vi "SeqMgr.Update Controls.vi"(8 "error in (no error)":errorcluster, 11 "SeqMgr in":refnum<class "SeqMgr.lvclass">) -> (0 "error out":errorcluster, 3 "SeqMgr out":refnum<class "SeqMgr.lvclass">)   [LabVIEW 2024, in "EQMF.lvlib" / "SeqMgr.lvlib" / "SeqMgr.lvclass"]
uses:
  SeqMgr.lvclass
  SeqMgr.lvclass/SeqMgr.ctl
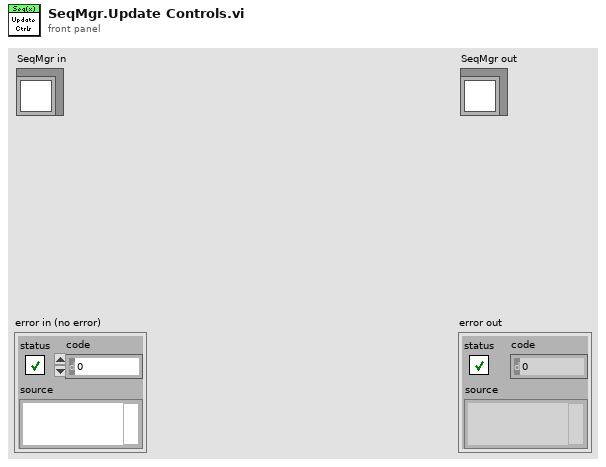
[diagram p1: front panel]
types:
  T1 = typedef "EQMF.lvlib/SeqMgr.lvlib/SeqMgr.Result State Enum.ctl" = enum16{"None", "Passing", "Failing", "PASS", "FAIL", "ABORT", "ERROR"}
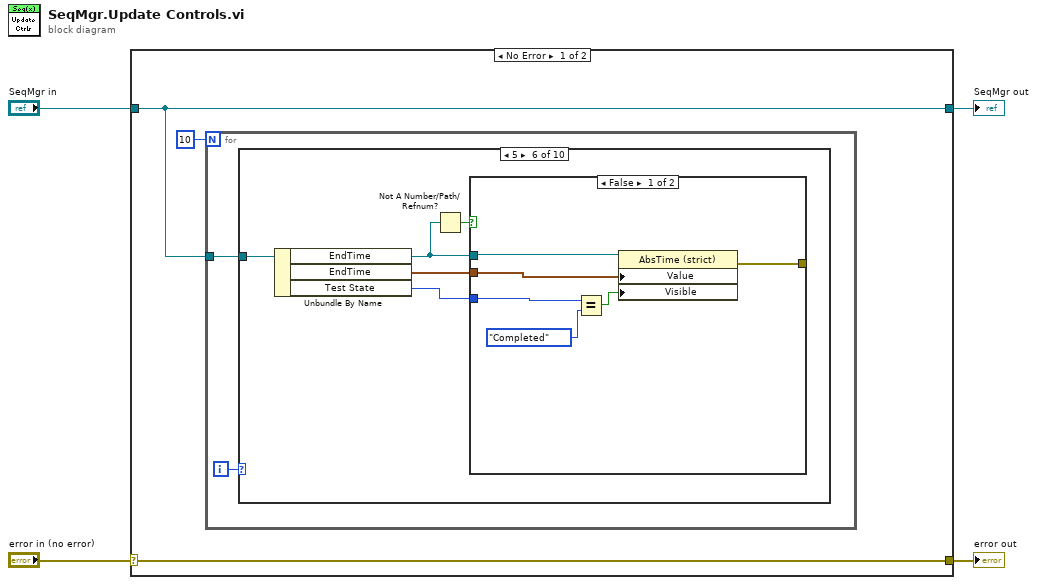
[diagram p0: block diagram]
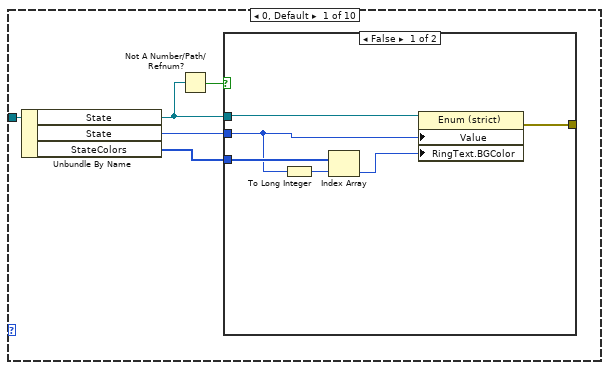
[diagram p2: hidden frame]
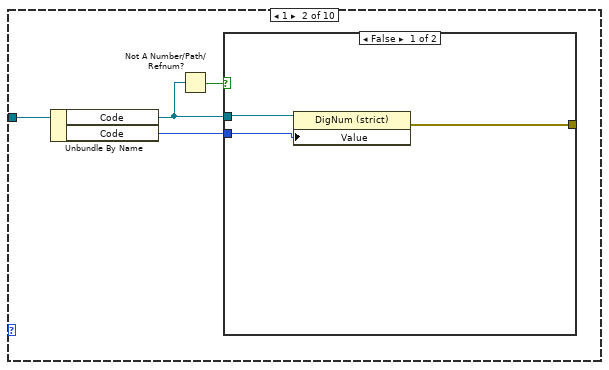
[diagram p4: hidden frame]
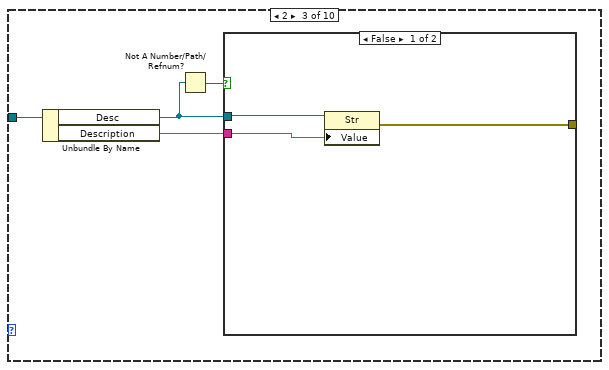
[diagram p6: hidden frame]
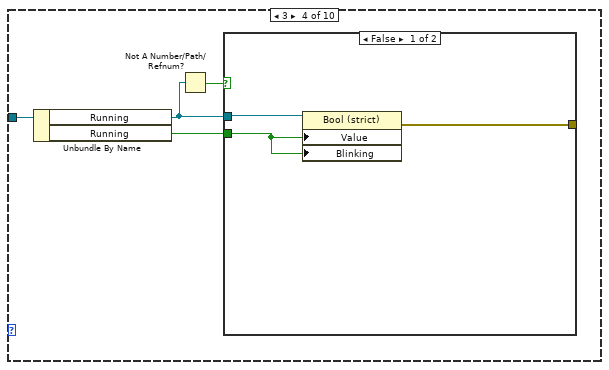
[diagram p8: hidden frame]
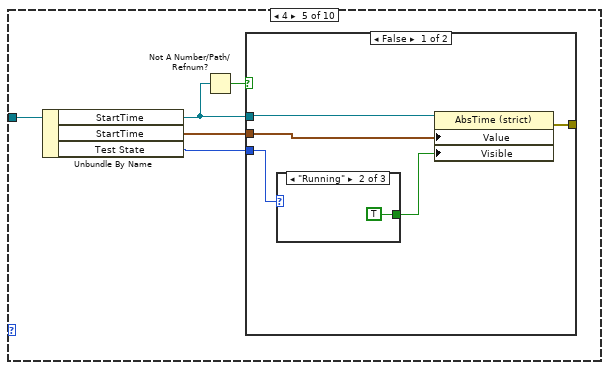
[diagram p10: hidden frame]
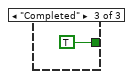
[diagram p12: hidden frame]
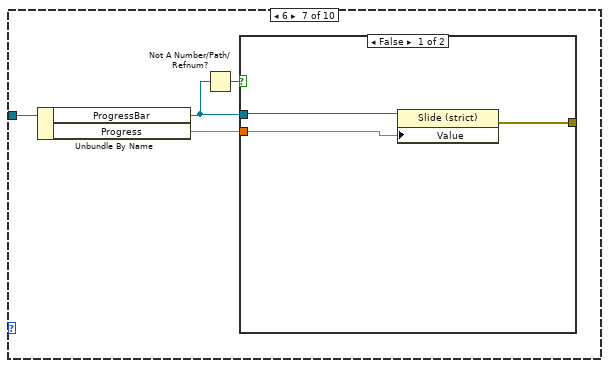
[diagram p15: hidden frame]
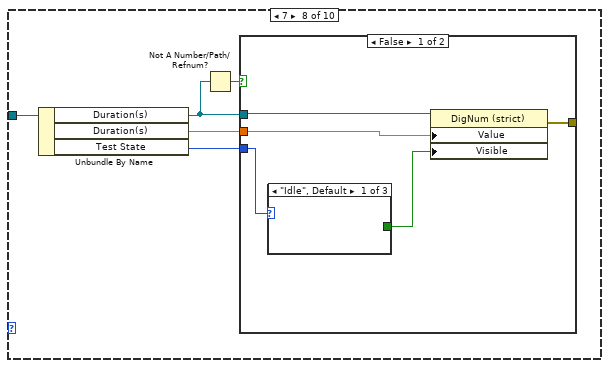
[diagram p17: hidden frame]
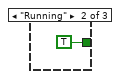
[diagram p18: hidden frame]
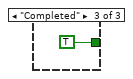
[diagram p19: hidden frame]
diagram:
  n1 = case shown="No Error" "error in (no error)" {
    selector: "error in (no error)" -> [w7 w104]
    tunnel: [w7 w104] -> w3
    tunnel: [w5 w103] -> w1
    tunnel: "SeqMgr in" -> [w5 w103]
    frame No Error {
      n2 = for {
        N: 10 -> [_]
        tunnel: w5 -> [w8]
        i -> [w9]
        n3 = case shown="5" w9 {
          tunnel: w8 -> [w13 w23 w30 w37 w45 w57 w67 w75 w86 w93]
          frame 0, Default {
            n4 = Unbundle By Name(w13) -> ("State"=w12:refnum<vi>, "State"=w11:T1, "StateColors"=w10:u32[])
            n5 = Not A Number/Path/Refnum?(number/path/refnum=w12) -> (NaN/Path/Refnum?=w14:bool)
            n6 = case shown="False" w14 {
              tunnel: w12 -> [w20 _]
              tunnel: w11 -> [w16 _]
              tunnel: [w19 _] -> _
              tunnel: w10 -> [w17 _]
              frame False {
                n7 = To Long Integer(number=w16) -> (32bit integer=w18:i32)
                n8 = Index Array(array=w17, index=w18) -> (element=w15:u32)
                n9 = property class="Enum (strict)"(reference=w20, "Value"=w16, "RingText.BGColor"=w15) -> (error out=w19:errorcluster)  [unwired: 1 in, 1 out]
              }
              frame True {
                # "Do nothing\nControl not configured"
              }
            }
          }
          frame 1 {
            n10 = Unbundle By Name(w23) -> ("Code"=w22:refnum<vi>, "Code"=w21:i32)
            n11 = Not A Number/Path/Refnum?(number/path/refnum=w22) -> (NaN/Path/Refnum?=w24:bool)
            n12 = case shown="False" w24 {
              tunnel: w22 -> [w27 _]
              tunnel: w21 -> [w26 _]
              tunnel: [w25 _] -> _
              frame False {
                n13 = property class="DigNum (strict)"(reference=w27, "Value"=w26) -> (error out=w25:errorcluster)  [unwired: 1 in, 1 out]
              }
              frame True {
                # "Do nothing\nControl not configured"
              }
            }
          }
          frame 2 {
            n14 = Unbundle By Name(w30) -> ("Desc"=w29:refnum<vi>, "Description"=w28:string)
            n15 = Not A Number/Path/Refnum?(number/path/refnum=w29) -> (NaN/Path/Refnum?=w31:bool)
            n16 = case shown="False" w31 {
              tunnel: w29 -> [w34 _]
              tunnel: w28 -> [w33 _]
              tunnel: [w32 _] -> _
              frame False {
                n17 = property class="Str"(reference=w34, "Value"=w33) -> (error out=w32:errorcluster)  [unwired: 1 in, 1 out]
              }
              frame True {
                # "Do nothing\nControl not configured"
              }
            }
          }
          frame 3 {
            n18 = Unbundle By Name(w37) -> ("Running"=w36:refnum<vi>, "Running"=w35:bool)
            n19 = Not A Number/Path/Refnum?(number/path/refnum=w36) -> (NaN/Path/Refnum?=w38:bool)
            n20 = case shown="False" w38 {
              tunnel: w36 -> [w41 _]
              tunnel: w35 -> [w39 _]
              tunnel: [w40 _] -> _
              frame False {
                n21 = property class="Bool (strict)"(reference=w41, "Value"=w39, "Blinking"=w39) -> (error out=w40:errorcluster)  [unwired: 1 in, 1 out]
              }
              frame True {
                # "Do nothing\nControl not configured"
              }
            }
          }
          frame 4 {
            n22 = Unbundle By Name(w45) -> ("StartTime"=w44:refnum<vi>, "StartTime"=w43:timestamp, "Test State"=w42:enum32{"Idle", "Running", "Completed"})
            n23 = Not A Number/Path/Refnum?(number/path/refnum=w44) -> (NaN/Path/Refnum?=w46:bool)
            n24 = case shown="False" w46 {
              tunnel: w44 -> [w51 _]
              tunnel: w43 -> [w50 _]
              tunnel: [w49 _] -> _
              tunnel: w42 -> [w48 _]
              frame False {
                n25 = case shown="\"Running\"" w48 {
                  tunnel: [_ TRUE TRUE] -> w47
                  frame "Idle", Default {
                  }
                  frame "Running" {
                  }
                  frame "Completed" {
                  }
                }
                n26 = property class="AbsTime (strict)"(reference=w51, "Value"=w50, "Visible"=w47) -> (error out=w49:errorcluster)  [unwired: 1 in, 1 out]
              }
              frame True {
                # "Do nothing\nControl not configured"
              }
            }
          }
          frame 5 {
            n27 = Unbundle By Name(w57) -> ("EndTime"=w56:refnum<vi>, "EndTime"=w54:timestamp, "Test State"=w55:enum32{"Idle", "Running", "Completed"})
            n28 = Not A Number/Path/Refnum?(number/path/refnum=w56) -> (NaN/Path/Refnum?=w58:bool)
            n29 = case shown="False" w58 {
              tunnel: w56 -> [w64 _]
              tunnel: w55 -> [w62 _]
              tunnel: [w63 _] -> _
              tunnel: w54 -> [w59 _]
              frame False {
                n30 = Equal?(x=w62, y=enum32{"Idle", "Running", "Completed"}."Completed") -> (x = y?=w60:bool)
                n31 = property class="AbsTime (strict)"(reference=w64, "Value"=w59, "Visible"=w60) -> (error out=w63:errorcluster)  [unwired: 1 in, 1 out]
              }
              frame True {
                # "Do nothing\nControl not configured"
              }
            }
          }
          frame 6 {
            n32 = Unbundle By Name(w67) -> ("ProgressBar"=w66:refnum<vi>, "Progress"=w65:dbl)
            n33 = Not A Number/Path/Refnum?(number/path/refnum=w66) -> (NaN/Path/Refnum?=w68:bool)
            n34 = case shown="False" w68 {
              tunnel: w66 -> [w71 _]
              tunnel: w65 -> [w69 _]
              tunnel: [w70 _] -> _
              frame False {
                n35 = property class="Slide (strict)"(reference=w71, "Value"=w69) -> (error out=w70:errorcluster)  [unwired: 1 in, 1 out]
              }
              frame True {
                # "Do nothing\nControl not configured"
              }
            }
          }
          frame 7 {
            n36 = Unbundle By Name(w75) -> ("Duration(s)"=w74:refnum<vi>, "Duration(s)"=w73:dbl, "Test State"=w72:enum32{"Idle", "Running", "Completed"})
            n37 = Not A Number/Path/Refnum?(number/path/refnum=w74) -> (NaN/Path/Refnum?=w76:bool)
            n38 = case shown="False" w76 {
              tunnel: w74 -> [w81 _]
              tunnel: w73 -> [w79 _]
              tunnel: [w80 _] -> _
              tunnel: w72 -> [w78 _]
              frame False {
                n39 = case shown="\"Idle\", Default" w78 {
                  tunnel: [_ TRUE TRUE] -> w77
                  frame "Idle", Default {
                  }
                  frame "Running" {
                  }
                  frame "Completed" {
                  }
                }
                n40 = property class="DigNum (strict)"(reference=w81, "Value"=w79, "Visible"=w77) -> (error out=w80:errorcluster)  [unwired: 1 in, 1 out]
              }
              frame True {
                # "Do nothing\nControl not configured"
              }
            }
          }
          frame 8 {
            n41 = Unbundle By Name(w86) -> ("Test Ctrl Tab"=w85:refnum<vi>, "Test State"=w84:enum32{"Idle", "Running", "Completed"})
            n42 = Not A Number/Path/Refnum?(number/path/refnum=w85) -> (NaN/Path/Refnum?=w87:bool)
            n43 = case shown="False" w87 {
              tunnel: w85 -> [w90 _]
              tunnel: w84 -> [w88 _]
              tunnel: [w89 _] -> _
              frame False {
                n44 = property class="TabCtl (strict)"(reference=w90, "Value"=w88) -> (error out=w89:errorcluster)  [unwired: 1 in, 1 out]
              }
              frame True {
                # "Do nothing\nControl not configured"
              }
            }
          }
          frame 9 {
            n45 = Unbundle By Name(w93) -> ("Failing Status"=w92:refnum<vi>, "State"=w91:T1)
            n46 = Not A Number/Path/Refnum?(number/path/refnum=w92) -> (NaN/Path/Refnum?=w94:bool)
            n47 = case shown="False" w94 {
              tunnel: w92 -> [w99 _]
              tunnel: w91 -> [w97 _]
              tunnel: [w98 _] -> _
              frame False {
                n48 = case shown="Default" w97 {
                  tunnel: ["" ("Value") "Failing" ("Value")] -> w96
                  tunnel: [_ TRUE] -> w95
                  frame Default {
                  }
                  frame "Failing" {
                  }
                }
                n49 = property class="Str"(reference=w99, "Value"=w96, "Visible"=w95) -> (error out=w98:errorcluster)  [unwired: 1 in, 1 out]
              }
              frame True {
                # "Do nothing\nControl not configured"
              }
            }
          }
        }
      }
    }
    frame Error {
    }
  }
  "error out" <- w3
  "SeqMgr out" <- w1
